vi "Hide File or Folder.vi"(8 "error in (no error)":errorcluster, 11 "File or Folder to Hide":path) -> (0 "error out":errorcluster, 2 "Operation Status":string)   [LabVIEW 2019, in "Tools.lvlib"]
doc: "This VI programatically hides <b>File or Folder to Hide</b>."
uses:
  Tools.lvlib
  kernel32.dll
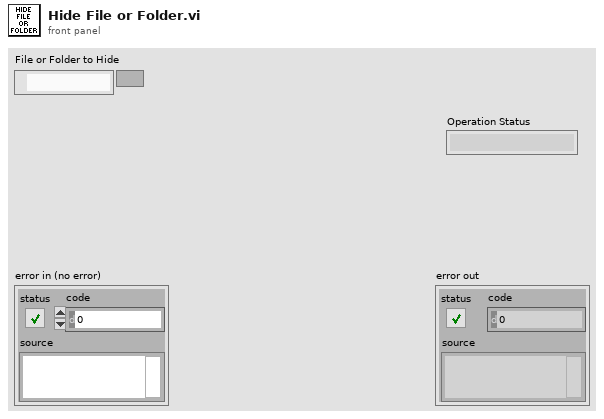
[diagram p1: front panel]
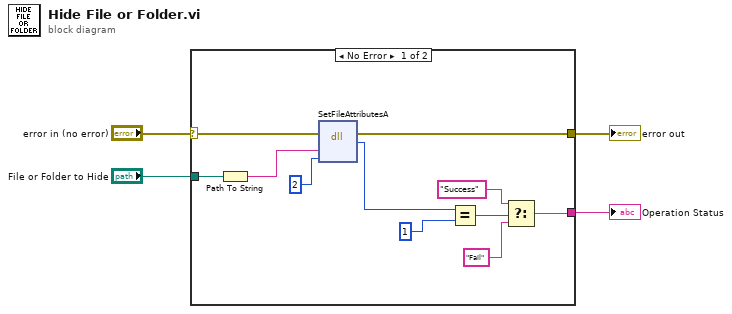
[diagram p0: block diagram]
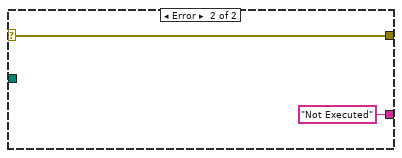
[diagram p2: hidden frame]
diagram:
  n1 = case shown="No Error" "error in (no error)" {
    selector: "error in (no error)" -> [w14 w17]
    tunnel: "File or Folder to Hide" -> [w13 _]
    tunnel: [w11 w17] -> w2
    tunnel: [w5 "Not Executed" ("Folder or File to Be Hidden")] -> w1
    frame No Error {
      n2 = Path To String(path=w13) -> (string=w12:string)
      n3 = dll-call lib="kernel32.dll" fn="SetFileAttributesA"(error in=w14, "lpFileName"=w12, "dwFileAttributes"=u32 2) -> (error out=w11:errorcluster, "return type"=w6:i32)  [unwired: 4 in, 1 out]
      n4 = Equal?(x=w6, y=1) -> (x = y?=w10:bool)
      n5 = Select(t="Success" ("Folder or File to Be Hidden"), s=w10, f="Fail" ("Folder or File to Be Hidden")) -> (s? t:f=w5:string)
    }
    frame Error {
    }
  }
  "error out" <- w2
  "Operation Status" <- w1
